vi "SendEventBack.vi"(8 "error in":errorcluster, 10 "error VIEW":errorcluster, 11 "CONTROLLER in":refnum<class "CONTROLLER.lvclass">) -> (0 "error out":errorcluster, 3 "CONTROLLER out":refnum<class "CONTROLLER.lvclass">)   [LabVIEW 2013, in "CONTROLLER.lvclass"]
uses:
  CONTROLLER.lvclass
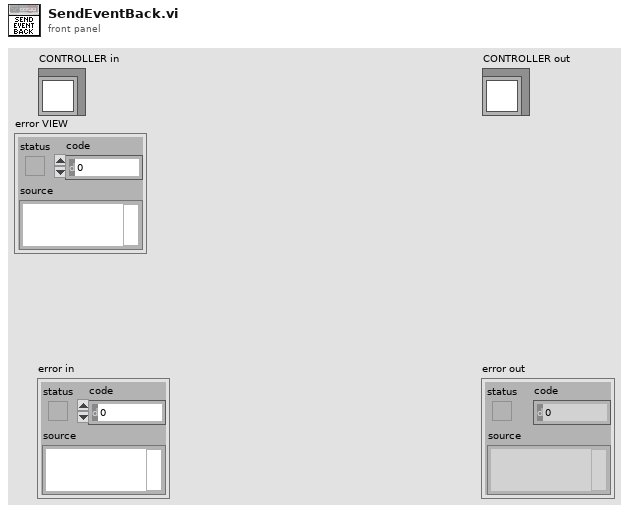
[diagram p1: front panel]
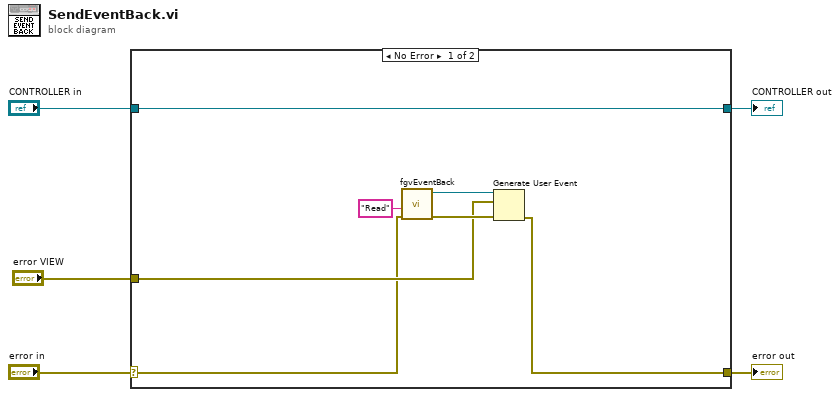
[diagram p0: block diagram]
diagram:
  n1 = case shown="No Error" "error in" {
    selector: "error in" -> [w7 w14]
    tunnel: [w6 w14] -> w4
    tunnel: [w12 w13] -> w2
    tunnel: "CONTROLLER in" -> [w12 w13]
    tunnel: "error VIEW" -> [w8 _]
    frame No Error {
      n2 = call "fgvEventBack.vi"("error in (no error)"=w7, "Cmd"="Read") -> ("error out"=w11:errorcluster, "EventData out"=w10:refnum<user-event>)  [unwired: 7 in, 1 out]
      n3 = Generate User Event(user event=w10, event data cluster=w8, error in=w11) -> (error out=w6:errorcluster)  [unwired: 1 in, 1 out]
    }
    frame Error {
    }
  }
  "error out" <- w4
  "CONTROLLER out" <- w2
